vi "WebDAV write.vi"(0 "RIO Filepath":path, 5 "CA Number":string, 7 "Test Name":string, 9 "Date":string, 11 "Filename":string) -> (15 "error out":errorcluster)   [LabVIEW 2013]
uses:
  <vilib>/WebDAVClient/Advanced/Put File.vi
  <vilib>/WebDAVClient/NI_WebDAV.lvlib
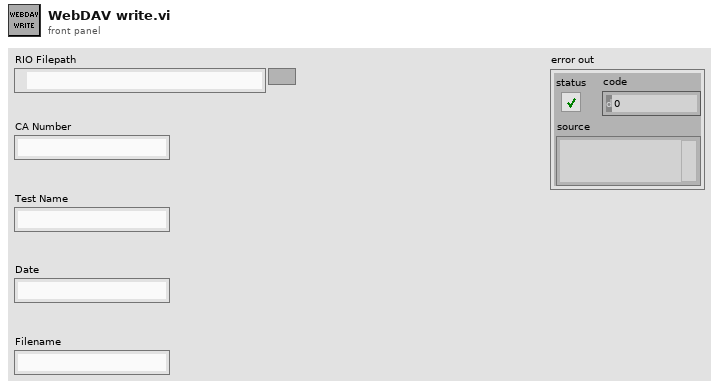
[diagram p1: front panel]
types:
  T1 = typedef "NI_WebDAV.lvlib/SessionHandle.ctl" = refnum<k1>
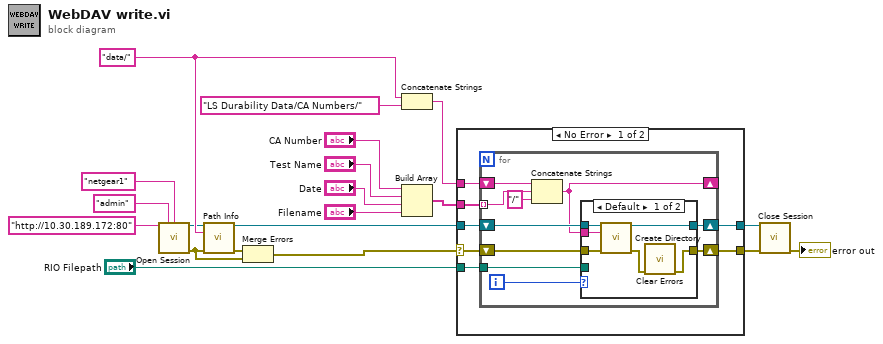
[diagram p0: block diagram]
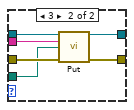
[diagram p2: hidden frame]
diagram:
  w19 = "data/" ("relative uri")
  n1 = call <vilib>:"Open Session.vi"("host uri prefix"="http://10.30.189.172:80", "username"="admin", "password"="netgear1") -> ("session handle out"=w13:T1, "error out"=w11:errorcluster)  [unwired: 11 in]
  n2 = call <vilib>:"Path Info.vi"("session handle"=w13, "relative uri"=w19, "error in (no error)"=w11) -> ("session handle out"=w14:T1, "error out"=w12:errorcluster)  [unwired: 9 in, 2 out]
  n3 = Merge Errors(w12, w11) -> (w16:errorcluster)
  n4 = Concatenate Strings(w19, "LS Durability Data/CA Numbers/" ("relative uri")) -> (w20:string)
  n5 = Build Array("CA Number", "Test Name", "Date", "Filename") -> (w5:string[])
  n6 = case shown="No Error" w16 {
    selector: w16 -> [w27 w51]
    tunnel: w14 -> [w26 w50]
    tunnel: [w23 w50] -> w15
    tunnel: [w22 w51] -> w17
    tunnel: w20 -> [w25 _]
    tunnel: w5 -> [w24 _]
    tunnel: "RIO Filepath" -> [w21 _]
    frame No Error {
      n7 = for {
        shift-right: [w32] -> _
        shift-left: w25 -> [w37]
        shift-right: [w33] -> w23
        shift-left: w26 -> [w34]
        shift-right: [w31] -> w22
        shift-left: w27 -> [w30]
        tunnel: w24 -> [w36] mode=indexing
        tunnel: w21 -> [w28]
        i -> [w29]
        n8 = Concatenate Strings(w37, w36, "/" ("string")) -> (w32:string)
        n9 = case shown="Default" w29 {
          tunnel: w34 -> [w43 w49]
          tunnel: [w42 w48] -> w33
          tunnel: w32 -> [w41 w47]
          tunnel: [w39 w45] -> w31
          tunnel: w30 -> [w38 w46]
          tunnel: w28 -> [_ w44]
          frame Default {
            n10 = call <vilib>:"Create Directory.vi"("session handle"=w43, "relative uri"=w41, "error in (no error)"=w38) -> ("session handle out"=w42:T1, "error out"=w40:errorcluster)  [unwired: 11 in]
            n11 = call <vilib>:"Clear Errors.vi"("error in (no error)"=w40) -> ("error out"=w39:errorcluster)  [unwired: 6 in]
          }
          frame 3 {
            n12 = call-poly <vilib>:"Put.vi"("session handle"=w49, "relative uri"=w47, "local file path"=w44, "error in (no error)"=w46) -> ("session handle out"=w48:T1, "error out"=w45:errorcluster)  [unwired: 9 in, 1 out]
          }
        }
      }
    }
    frame Error {
    }
  }
  n13 = call <vilib>:"Close Session.vi"("session handle"=w15, "error in (no error)"=w17) -> ("error out"=→"error out":errorcluster)  [unwired: 13 in]
